vi "Front Panel Tyler.vi"() -> ()   [LabVIEW 2017, in "LD Reading.lvclass"]
uses:
  LD Reading.lvclass
  Reference Channel Intensities.ctl
  Sample Channel Intensities.ctl
  Realtime Output.ctl
  LD Reading.lvclass/LD Reading.ctl
  <vilib>/Analysis/baseanly.llb/Mean (DBL).vi
  <vilib>/Utility/file.llb/Write Delimited Spreadsheet (DBL).vi
  <vilib>/Analysis/NI_AALBase.lvlib
panel:
  out "Data Collection Progress":u8(slide) scale=0.0..100.0
  out "Current Phase":string
  in  "Data graphs":enum32{"Data", "Miscellaneous Data"}(tab)
  out "Diode/PMT":cluster{dbl[], dbl[]}(graph)
  out "RMS Voltage (mV)":cluster{dbl[], dbl[]}(graph)
  out "Photodiode Voltage  (V)":cluster{dbl[], dbl[]}(graph)
  out "PMT Voltage (V)":cluster{dbl[], dbl[]}(graph)
  in  "Data Collection Mode":enum32{"Reference", "Sample"}(radio)
  in  "Selected Sample Channel":enum32{"Channel 1", "Channel 2", "Channel 3"}(radio)
  in  "Selected Reference Channel":enum32{"Channel 1", "Channel 2", "Channel 3"}(radio)
  out "Realtime Output":T1
  out "Sample Data":T2
  out "Reference Data":T3
  in  "Correction Factor":dbl
  out "Finished":bool
  in  "Output Filename (stem)":path
  in  "Stop Data Collection":bool
  in  "Save Data?":bool
  out "Running":bool
  in  "Number of Data Points":dbl
  in  "Data Interval (s)":dbl
  in  "Collect Data":bool
  in  "stop":bool
  # "Data Collection Parameters"
  # "Experiment Control"
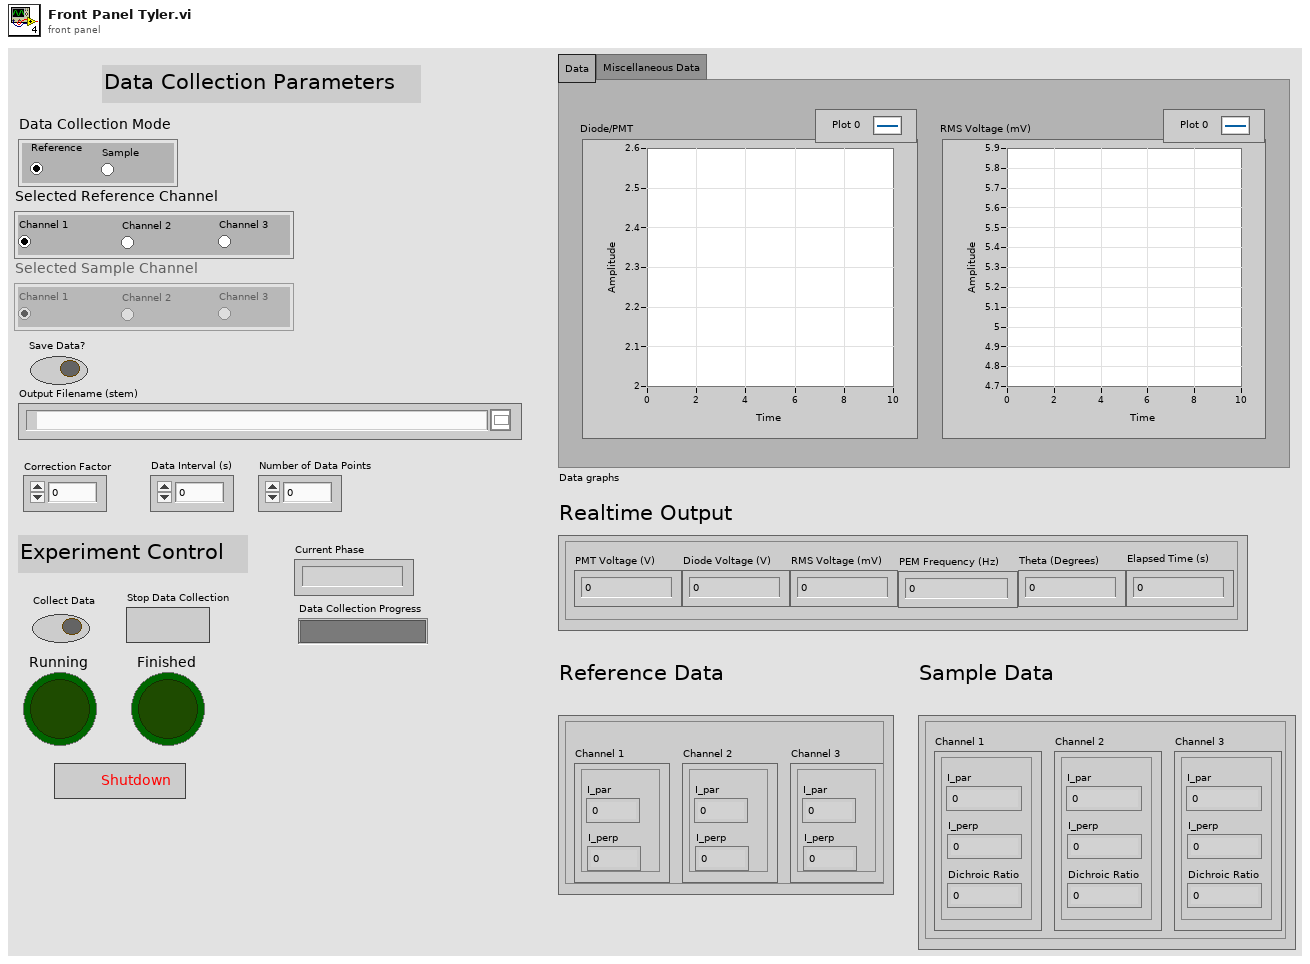
[diagram p1: front panel]
types:
  T1 = typedef "Realtime Output.ctl" = cluster{"Elapsed Time (s)":dbl, "PMT Voltage (V)":dbl, "Diode Voltage (V)":dbl, "RMS Voltage (mV)":dbl, "Theta (Degrees)":dbl, "PEM Frequency (Hz)":dbl}
  T2 = typedef "Sample Channel Intensities.ctl" = cluster{"Channel 1":cluster{"I_par":dbl, "I_perp":dbl, "Dichroic Ratio":dbl}, "Channel 2":cluster{"I_par":dbl, "I_perp":dbl, "Dichroic Ratio":dbl}, "Channel 3":cluster{"I_par":dbl, "I_perp":dbl, "Dichroic Ratio":dbl}}
  T3 = typedef "Reference Channel Intensities.ctl" = cluster{"Channel 1":cluster{"I_par":dbl, "I_perp":dbl}, "Channel 2":cluster{"I_par":dbl, "I_perp":dbl}, "Channel 3":cluster{"I_par":dbl, "I_perp":dbl}}
  T4 = enum8{"Enabled", "Disabled", "Disabled and Grayed Out"}
  T5 = cluster{"I_par":dbl, "I_perp":dbl, "Dichroic Ratio":dbl}
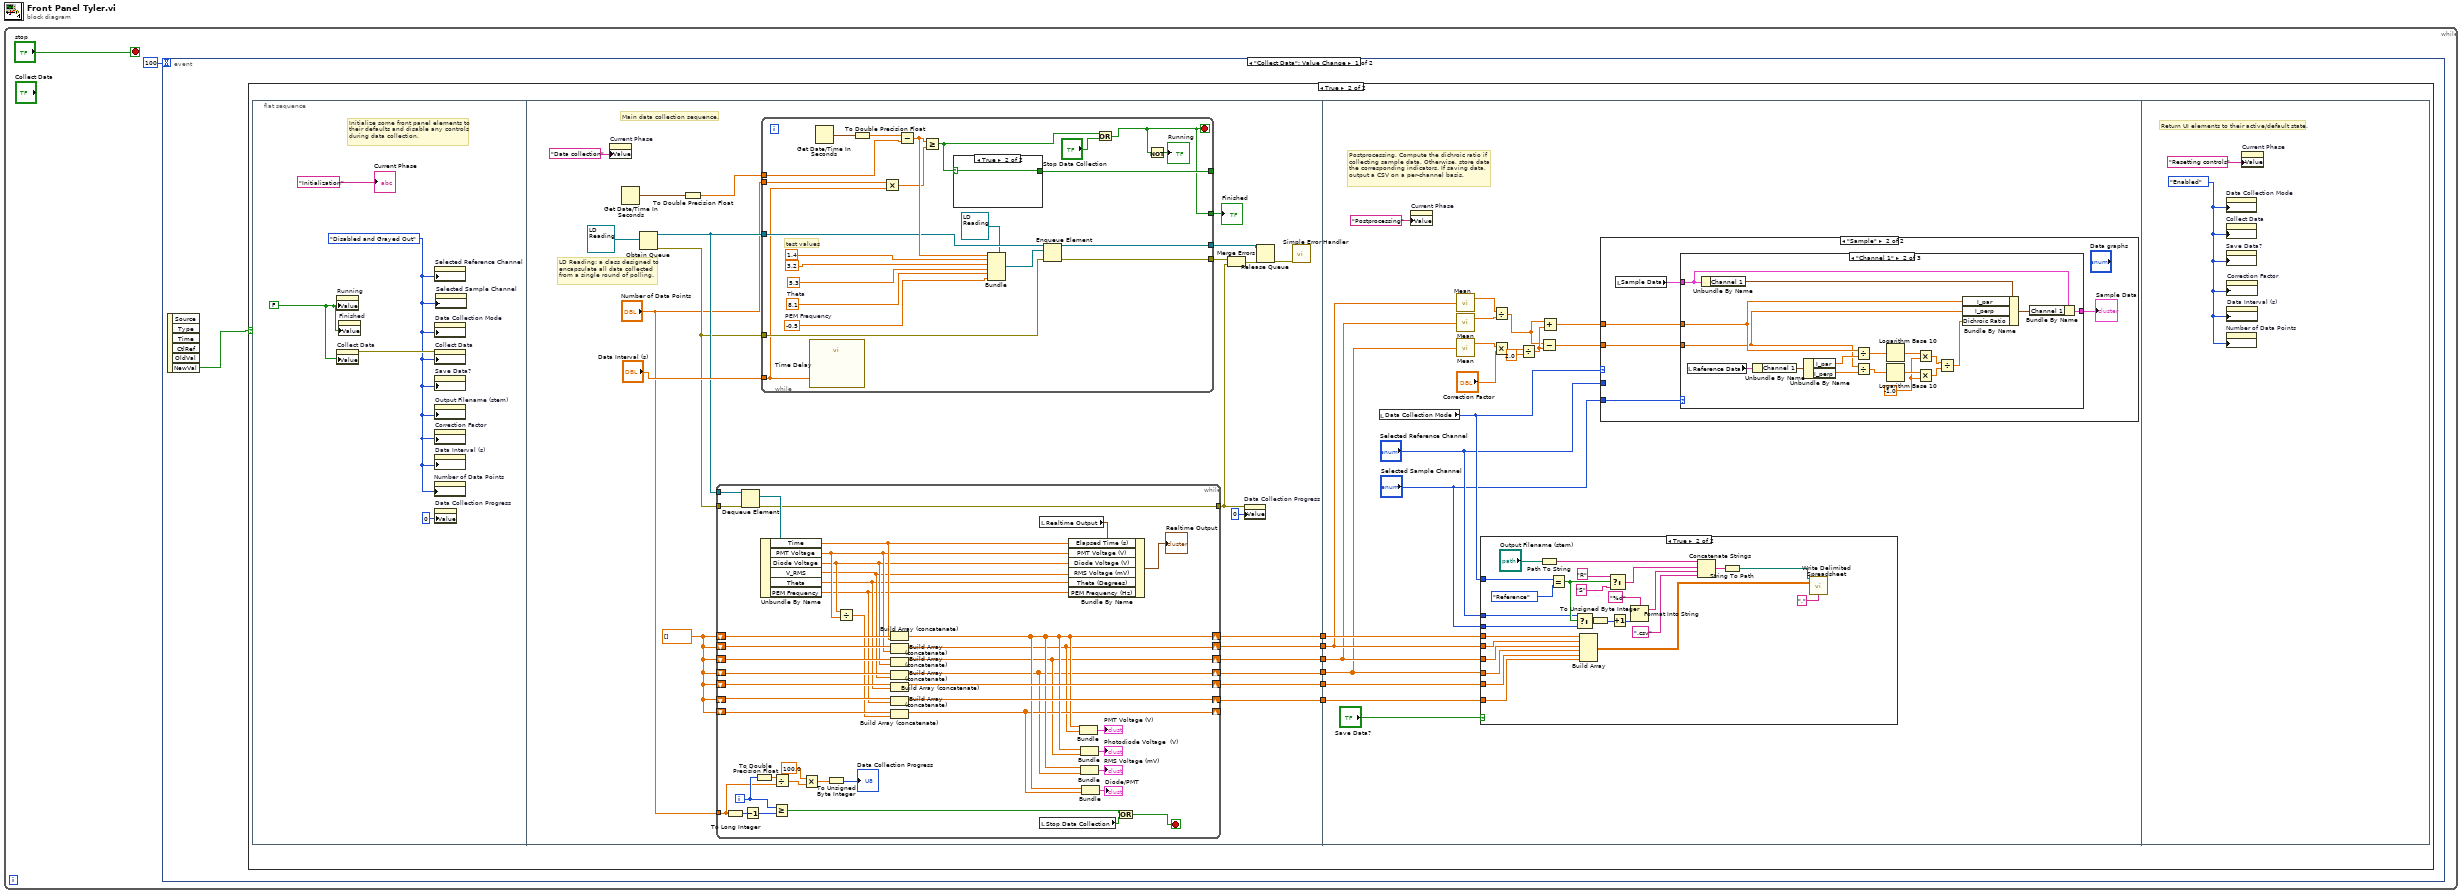
[diagram p0: block diagram]
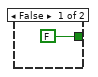
[diagram p3: hidden frame]
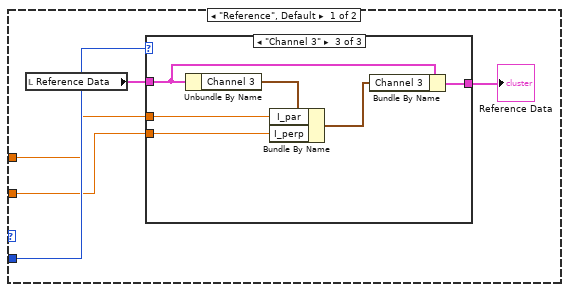
[diagram p5: hidden frame]
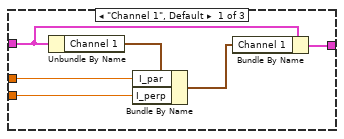
[diagram p6: hidden frame]
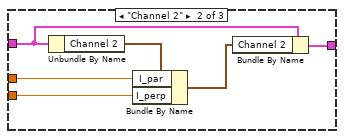
[diagram p7: hidden frame]
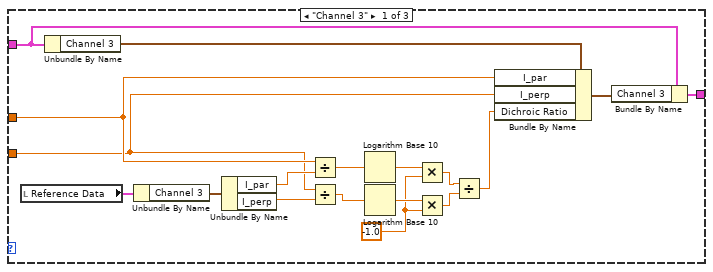
[diagram p8: hidden frame]
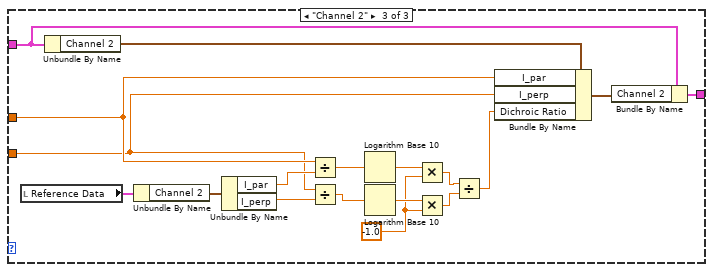
[diagram p9: hidden frame]
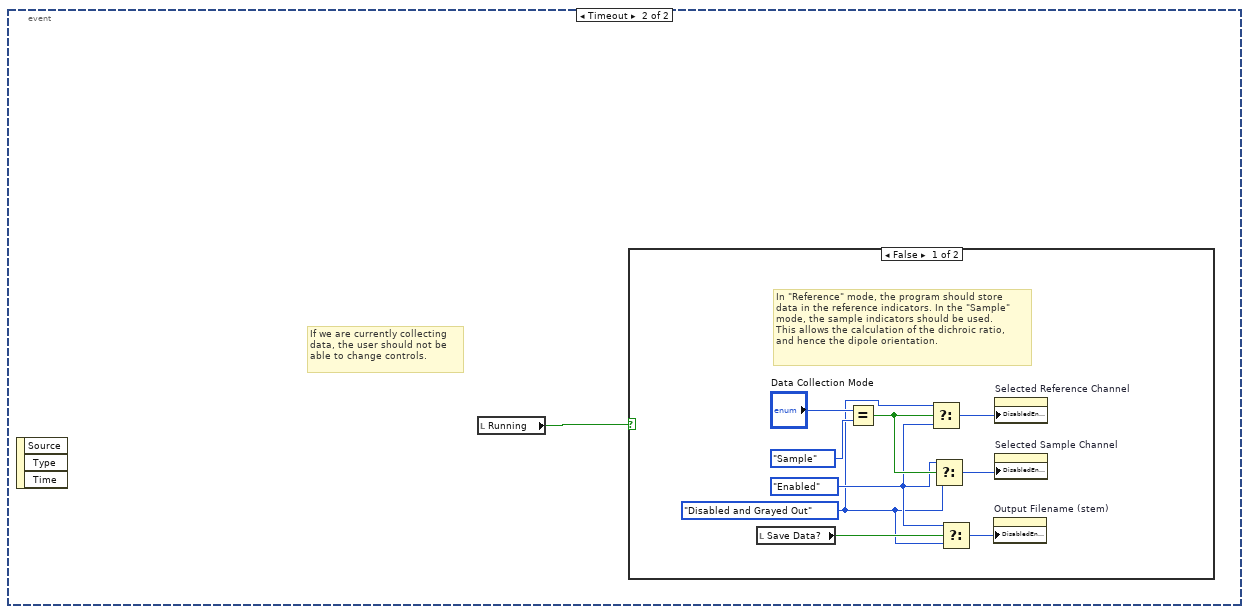
[diagram p10: hidden frame]
diagram:
  n1 = while {
    stop <- "stop" stop-if-true
    n2 = event shown="[0] \"Collect Data\": Value Change" {
      selector: _ -> [_ _]
      dyn-events: _ -> [_ _]
      timeout: 100 -> [_ _]
      event "Collect Data": Value Change {
        n3 = event-data() -> ("NewVal"=w3:bool)  [unwired: 1 in, 5 out]
        n4 = case shown="True" w3 {
          frame False {
          }
          frame True {
            n5 = flat-sequence {
              tunnel: [w23] -> w9
              tunnel: [w22] -> w8
              tunnel: [w21] -> w7
              tunnel: [w24] -> w6
              tunnel: [w20] -> w5
              tunnel: [w19] -> w4
              tunnel: w9 -> [w108]
              tunnel: w8 -> [w107]
              tunnel: w7 -> [w106]
              tunnel: w6 -> [w114]
              tunnel: w5 -> [w110]
              tunnel: w4 -> [w109]
              frame #0 {
                w12 = T4."Disabled and Grayed Out" ("Disabled")
                w14 = FALSE
                # "Initialize some front panel elements to \ntheir defaults and disable any controls \nduring data collection."
                n6 = property on="Running" class="Bool (strict)"("Value"=w14) -> ()  [unwired: 2 in, 2 out]
                n7 = property on="Collect Data" class="Bool (strict)"("Value"=w14) -> (error out=w13:errorcluster)  [unwired: 2 in, 1 out]
                n8 = property on="Finished" class="Bool (strict)"("Value"=w14) -> ()  [unwired: 2 in, 2 out]
                n9 = property on="Number of Data Points" class="DigNum (strict)"("DisabledEnum"=w12) -> ()  [unwired: 2 in, 2 out]
                n10 = property on="Selected Reference Channel" class="RadioBtnsControl (strict)"("DisabledEnum"=w12) -> ()  [unwired: 2 in, 2 out]
                n11 = property on="Data Collection Mode" class="RadioBtnsControl (strict)"("DisabledEnum"=w12) -> ()  [unwired: 2 in, 2 out]
                n12 = property on="Collect Data" class="Bool (strict)"(error in=w13, "DisabledEnum"=w12) -> ()  [unwired: 1 in, 2 out]
                n13 = property on="Save Data?" class="Bool (strict)"("DisabledEnum"=w12) -> ()  [unwired: 2 in, 2 out]
                n14 = property on="Output Filename (stem)" class="Path"("DisabledEnum"=w12) -> ()  [unwired: 2 in, 2 out]
                n15 = property on="Correction Factor" class="DigNum (strict)"("DisabledEnum"=w12) -> ()  [unwired: 2 in, 2 out]
                n16 = property on="Data Interval (s)" class="DigNum (strict)"("DisabledEnum"=w12) -> ()  [unwired: 2 in, 2 out]
                n17 = property on="Data Collection Progress" class="Slide (strict)"("Value"=u8 0 ("Progress")) -> ()  [unwired: 2 in, 2 out]
                n18 = property on="Selected Sample Channel" class="RadioBtnsControl (strict)"("DisabledEnum"=w12) -> ()  [unwired: 2 in, 2 out]
                "Current Phase" <- "Initialization"
              }
              frame #1 {
                w18 = dbl[] []
                # "Main data collection sequence."
                # "LD Reading: a class designed to \nencapsulate all data collected \nfrom a single round of polling."
                n19 = property on="Current Phase" class="Str"("Value"="Data collection") -> ()  [unwired: 2 in, 2 out]
                n20 = Get Date/Time In Seconds() -> (seconds since 1Jan1904=w35:timestamp)
                n21 = Obtain Queue(element data type=refnum<class "LD Reading.lvclass"> refnum ("LD Reading.lvclass")) -> (queue out=w32:refnum<queue>, error out=w30:errorcluster)  [unwired: 4 in, 1 out]
                n22 = To Double Precision Float(number=w35) -> (double precision float=w34:dbl)
                n23 = while {
                  tunnel: w32 -> [w79]
                  shift-right: [w65] -> w24
                  shift-left: w18 -> [w75]
                  shift-right: [w59] -> w23
                  shift-left: w18 -> [w74]
                  shift-right: [w58] -> w22
                  shift-left: w18 -> [w72]
                  shift-right: [w57] -> w21
                  shift-left: w18 -> [w71]
                  shift-right: [w69] -> w20
                  shift-left: w18 -> [w70]
                  shift-right: [w67] -> w19
                  shift-left: w18 -> [w68]
                  shift-right: [w62] -> _
                  shift-left: w18 -> [w64]
                  tunnel: w30 -> [w56]
                  tunnel: [w55] -> w16
                  tunnel: "Number of Data Points" -> [w41]
                  i -> [w42]
                  stop <- w77 stop-if-true
                  n24 = To Long Integer(number=w41) -> (32bit integer=w43:i32)
                  n25 = Dequeue Element(queue=w79, error in (no error)=w56) -> (element=w78:refnum<class "LD Reading.lvclass">, error out=w55:errorcluster)  [unwired: 1 in, 2 out]
                  n26 = Decrement(x=w43) -> (x-1=w54:i32)
                  n27 = To Double Precision Float(number=w42) -> (double precision float=w40:dbl)
                  n28 = Unbundle By Name(w78) -> ("Time"=w51:dbl, "PMT Voltage"=w50:dbl, "Diode Voltage"=w49:dbl, "V_RMS"=w48:dbl, "Theta"=w47:dbl, "PEM Frequency"=w46:dbl)
                  n29 = Greater Or Equal?(x=w42, y=w54) -> (x >= y?=w53:bool)
                  n30 = Divide(x=w40, y=w41) -> (x/y=w44:dbl)
                  n31 = Multiply(x=100.0, y=w44) -> (x*y=w38:dbl)
                  n32 = To Unsigned Byte Integer(number=w38) -> (unsigned 8bit integer=→"Data Collection Progress":u8)
                  n33 = Divide(x=w49, y=w50) -> (x/y=w63:dbl)
                  n34 = Build Array (concatenate)(w75, w51) -> (w65:dbl[])
                  n35 = Build Array (concatenate)(w74, w50) -> (w59:dbl[])
                  n36 = Build Array (concatenate)(w72, w49) -> (w58:dbl[])
                  n37 = Build Array (concatenate)(w71, w48) -> (w57:dbl[])
                  n38 = Build Array (concatenate)(w70, w47) -> (w69:dbl[])
                  n39 = Build Array (concatenate)(w68, w46) -> (w67:dbl[])
                  n40 = Build Array (concatenate)(w64, w63) -> (w62:dbl[])
                  n41 = local read "Realtime Output"() -> (w45:T1)
                  n42 = local read "Stop Data Collection"() -> (w76:bool)
                  n43 = Bundle By Name(cluster=w45, "Elapsed Time (s)"=w51, "PMT Voltage (V)"=w50, "Diode Voltage (V)"=w49, "RMS Voltage (mV)"=w48, "Theta (Degrees)"=w47, "PEM Frequency (Hz)"=w46) -> (→"Realtime Output":T1)
                  n44 = Bundle(w65, w59) -> (→"PMT Voltage (V)":cluster{dbl[], dbl[]})  [unwired: 1 in]
                  n45 = Bundle(w65, w58) -> (→"Photodiode Voltage  (V)":cluster{dbl[], dbl[]})  [unwired: 1 in]
                  n46 = Bundle(w65, w57) -> (→"RMS Voltage (mV)":cluster{dbl[], dbl[]})  [unwired: 1 in]
                  n47 = Bundle(w65, w62) -> (→"Diode/PMT":cluster{dbl[], dbl[]})  [unwired: 1 in]
                  n48 = Or(x=w53, y=w76) -> (x .or. y?=w77:bool)
                }
                n49 = while {
                  tunnel: "Data Interval (s)" -> [w82]
                  tunnel: w34 -> [w83]
                  tunnel: [w99] -> _
                  tunnel: w32 -> [w92]
                  tunnel: [w89] -> w26
                  tunnel: [w86] -> w31
                  tunnel: w30 -> [w85]
                  tunnel: [w84] -> w29
                  tunnel: "Number of Data Points" -> [w81]
                  stop <- w86 stop-if-true
                  w93 = -0.5  # PEM Frequency
                  w94 = 8.1  # Theta
                  # "test values"
                  n50 = call "Time Delay"("Delay Time (s)"=w82) -> ()  [unwired: 10 in, 1 out]
                  n51 = Get Date/Time In Seconds() -> (seconds since 1Jan1904=w102:timestamp)
                  n52 = To Double Precision Float(number=w102) -> (double precision float=w101:dbl)
                  n53 = Multiply(x=w81, y=w82) -> (x*y=w80:dbl)
                  n54 = Subtract(x=w101, y=w83) -> (x-y=w96:dbl)
                  n55 = Greater Or Equal?(x=w96, y=w80) -> (x >= y?=w87:bool)
                  n56 = case shown="True" w87 {
                    selector: w87 -> [_ w104]
                    tunnel: [FALSE w104] -> w99
                    frame False {
                    }
                    frame True {
                    }
                  }
                  n57 = Bundle(cluster=refnum<class "LD Reading.lvclass"> refnum ("LD Reading.lvclass"), w96, 1.4 ("PMT Voltage"), 3.2 ("Diode Voltage"), 5.3 ("V_RMS"), w94, w93) -> (w90:refnum<class "LD Reading.lvclass">)
                  n58 = Enqueue Element(queue=w92, element=w90, error in (no error)=w85) -> (queue out=w89:refnum<queue>, error out=w84:errorcluster)  [unwired: 1 in, 1 out]
                  n59 = Or(x=w87, y="Stop Data Collection") -> (x .or. y?=w86:bool)
                  n60 = Not(x=w86) -> (.not. x?=→"Running":bool)
                }
                "Finished" <- w31
                n61 = Merge Errors(w29, w16) -> (w28:errorcluster)
                n62 = property on="Data Collection Progress" class="Slide (strict)"(error in=w16, "Value"=u8 0 ("Progress")) -> ()  [unwired: 1 in, 2 out]
                n63 = Release Queue(queue=w26, error in (no error)=w28) -> (error out=w27:errorcluster)  [unwired: 1 in, 2 out]
                n64 = call <vilib>:"Simple Error Handler.vi"("error in (no error)"=w27) -> ()  [unwired: 4 in, 5 out]
              }
              frame #2 {
                # "Postprocessing. Compute the dichroic ratio if \ncollecting sample data. Otherwise, store data \nthe corresponding indicators. If saving data, \noutput a CSV on a per-channel basis."
                n65 = local read "Data Collection Mode"() -> (w113:enum32{"Reference", "Sample"})
                n66 = property on="Current Phase" class="Str"("Value"="Postprocessing") -> ()  [unwired: 2 in, 2 out]
                n67 = call-poly <vilib>:"Mean.vi"("X"=w108) -> ("mean"=w118:dbl)  [unwired: 1 out]
                n68 = call-poly <vilib>:"Mean.vi"("X"=w107) -> ("mean"=w117:dbl)  [unwired: 1 out]
                n69 = call-poly <vilib>:"Mean.vi"("X"=w106) -> ("mean"=w124:dbl)  [unwired: 1 out]
                n70 = case shown="True" "Save Data?" {
                  tunnel: w106 -> [_ w133]
                  tunnel: w107 -> [_ w134]
                  tunnel: w108 -> [_ w135]
                  tunnel: w114 -> [_ w136]
                  tunnel: w113 -> [_ w151]
                  tunnel: "Selected Reference Channel" -> [_ w146]
                  tunnel: "Selected Sample Channel" -> [_ w145]
                  tunnel: w110 -> [_ w127]
                  tunnel: w109 -> [_ w126]
                  frame False {
                  }
                  frame True {
                    n71 = Path To String(path="Output Filename (stem)") -> (string=w143:string)
                    n72 = Equal?(x=w151, y=enum32{"Reference", "Sample"}."Reference" ("Data Collection Mode")) -> (x = y?=w147:bool)
                    n73 = Select(t=w146, s=w147, f=w145) -> (s? t:f=w142:enum32{"Channel 1", "Channel 2", "Channel 3"})
                    n74 = Build Array(w136, w135, w134, w133, w127, w126) -> (w132:dbl[][])
                    n75 = To Unsigned Byte Integer(number=w142) -> (unsigned 8bit integer=w130:u8)
                    n76 = Select(t="R", s=w147, f="S") -> (s? t:f=w140:string)
                    n77 = Increment(x=w130) -> (x+1=w129:u8)
                    n78 = Format Into String(format string="%d", w129) -> (resulting string=w139:string)  [unwired: 2 in, 1 out]
                    n79 = Concatenate Strings(w143, w140, w139, ".csv" ("string")) -> (w137:string)
                    n80 = String To Path(string=w137) -> (path=w131:path)
                    n81 = call-poly <vilib>:"Write Delimited Spreadsheet.vi"("file path (dialog if empty)"=w131, "2D data"=w132, "delimiter (\\t)"="," ("delimiter (\\t)")) -> ()  [unwired: 11 in, 2 out]
                  }
                }
                n82 = Divide(x=w118, y=w117) -> (x/y=w116:dbl)
                n83 = Multiply(x=w124, y="Correction Factor") -> (x*y=w123:dbl)
                n84 = Divide(x=w123, y=2.0) -> (x/y=w121:dbl)
                n85 = Subtract(x=w116, y=w121) -> (x-y=w119:dbl)
                n86 = Add(x=w116, y=w121) -> (x+y=w120:dbl)
                n87 = case shown="\"Sample\"" w113 {
                  tunnel: "Selected Reference Channel" -> [w156 _]
                  tunnel: w120 -> [w155 w179]
                  tunnel: w119 -> [w154 w178]
                  tunnel: "Selected Sample Channel" -> [_ w176]
                  frame "Reference", Default {
                    n88 = local read "Reference Data"() -> (w153:T3)
                    n89 = case shown="\"Channel 3\"" w156 {
                      tunnel: w155 -> [w161 w167 w173]
                      tunnel: w154 -> [w160 w166 w172]
                      tunnel: w153 -> [w159 w165 w171]
                      tunnel: [w157 w163 w169] -> w152
                      frame "Channel 1", Default {
                        n90 = Unbundle By Name(w159) -> ("Channel 1"=w162:cluster{"I_par":dbl, "I_perp":dbl})
                        n91 = Bundle By Name(cluster=w162, "I_par"=w161, "I_perp"=w160) -> (w158:cluster{"I_par":dbl, "I_perp":dbl})
                        n92 = Bundle By Name(cluster=w159, "Channel 1"=w158) -> (w157:T3)
                      }
                      frame "Channel 2" {
                        n93 = Unbundle By Name(w165) -> ("Channel 2"=w168:cluster{"I_par":dbl, "I_perp":dbl})
                        n94 = Bundle By Name(cluster=w168, "I_par"=w167, "I_perp"=w166) -> (w164:cluster{"I_par":dbl, "I_perp":dbl})
                        n95 = Bundle By Name(cluster=w165, "Channel 2"=w164) -> (w163:T3)
                      }
                      frame "Channel 3" {
                        n96 = Unbundle By Name(w171) -> ("Channel 3"=w174:cluster{"I_par":dbl, "I_perp":dbl})
                        n97 = Bundle By Name(cluster=w174, "I_par"=w173, "I_perp"=w172) -> (w170:cluster{"I_par":dbl, "I_perp":dbl})
                        n98 = Bundle By Name(cluster=w171, "Channel 3"=w170) -> (w169:T3)
                      }
                    }
                    "Reference Data" <- w152
                  }
                  frame "Sample" {
                    n99 = local read "Sample Data"() -> (w177:T2)
                    n100 = case shown="\"Channel 1\"" w176 {
                      tunnel: w179 -> [w186 w204 w222]
                      tunnel: w178 -> [w185 w203 w221]
                      tunnel: w177 -> [w182 w200 w218]
                      tunnel: [w180 w198 w216] -> w175
                      frame "Channel 3" {
                        w189 = -1.0
                        n101 = local read "Reference Data"() -> (w197:T3)
                        n102 = Unbundle By Name(w182) -> ("Channel 3"=w184:T5)
                        n103 = Unbundle By Name(w197) -> ("Channel 3"=w196:cluster{"I_par":dbl, "I_perp":dbl})
                        n104 = Unbundle By Name(w196) -> ("I_par"=w195:dbl, "I_perp"=w194:dbl)
                        n105 = Divide(x=w186, y=w195) -> (x/y=w192:dbl)
                        n106 = Divide(x=w185, y=w194) -> (x/y=w193:dbl)
                        n107 = Logarithm Base 10(1:w192) -> (0:w190:dbl)
                        n108 = Logarithm Base 10(1:w193) -> (0:w191:dbl)
                        n109 = Multiply(x=w190, y=w189) -> (x*y=w187:dbl)
                        n110 = Multiply(x=w191, y=w189) -> (x*y=w188:dbl)
                        n111 = Divide(x=w187, y=w188) -> (x/y=w183:dbl)
                        n112 = Bundle By Name(cluster=w184, "I_par"=w186, "I_perp"=w185, "Dichroic Ratio"=w183) -> (w181:T5)
                        n113 = Bundle By Name(cluster=w182, "Channel 3"=w181) -> (w180:T2)
                      }
                      frame "Channel 1" {
                        w207 = -1.0
                        n114 = local read "Reference Data"() -> (w215:T3)
                        n115 = Unbundle By Name(w200) -> ("Channel 1"=w202:T5)
                        n116 = Unbundle By Name(w215) -> ("Channel 1"=w214:cluster{"I_par":dbl, "I_perp":dbl})
                        n117 = Unbundle By Name(w214) -> ("I_par"=w213:dbl, "I_perp"=w212:dbl)
                        n118 = Divide(x=w204, y=w213) -> (x/y=w210:dbl)
                        n119 = Divide(x=w203, y=w212) -> (x/y=w211:dbl)
                        n120 = Logarithm Base 10(1:w210) -> (0:w208:dbl)
                        n121 = Logarithm Base 10(1:w211) -> (0:w209:dbl)
                        n122 = Multiply(x=w208, y=w207) -> (x*y=w205:dbl)
                        n123 = Multiply(x=w209, y=w207) -> (x*y=w206:dbl)
                        n124 = Divide(x=w205, y=w206) -> (x/y=w201:dbl)
                        n125 = Bundle By Name(cluster=w202, "I_par"=w204, "I_perp"=w203, "Dichroic Ratio"=w201) -> (w199:T5)
                        n126 = Bundle By Name(cluster=w200, "Channel 1"=w199) -> (w198:T2)
                      }
                      frame "Channel 2" {
                        w225 = -1.0
                        n127 = local read "Reference Data"() -> (w233:T3)
                        n128 = Unbundle By Name(w218) -> ("Channel 2"=w220:T5)
                        n129 = Unbundle By Name(w233) -> ("Channel 2"=w232:cluster{"I_par":dbl, "I_perp":dbl})
                        n130 = Unbundle By Name(w232) -> ("I_par"=w231:dbl, "I_perp"=w230:dbl)
                        n131 = Divide(x=w222, y=w231) -> (x/y=w228:dbl)
                        n132 = Divide(x=w221, y=w230) -> (x/y=w229:dbl)
                        n133 = Logarithm Base 10(1:w228) -> (0:w226:dbl)
                        n134 = Logarithm Base 10(1:w229) -> (0:w227:dbl)
                        n135 = Multiply(x=w226, y=w225) -> (x*y=w223:dbl)
                        n136 = Multiply(x=w227, y=w225) -> (x*y=w224:dbl)
                        n137 = Divide(x=w223, y=w224) -> (x/y=w219:dbl)
                        n138 = Bundle By Name(cluster=w220, "I_par"=w222, "I_perp"=w221, "Dichroic Ratio"=w219) -> (w217:T5)
                        n139 = Bundle By Name(cluster=w218, "Channel 2"=w217) -> (w216:T2)
                      }
                    }
                    "Sample Data" <- w175
                  }
                }
              }
              frame #3 {
                w235 = T4."Enabled" ("Disabled")
                # "Return UI elements to their active/default state."
                n140 = property on="Data Collection Mode" class="RadioBtnsControl (strict)"("DisabledEnum"=w235) -> ()  [unwired: 2 in, 2 out]
                n141 = property on="Collect Data" class="Bool (strict)"("DisabledEnum"=w235) -> ()  [unwired: 2 in, 2 out]
                n142 = property on="Save Data?" class="Bool (strict)"("DisabledEnum"=w235) -> ()  [unwired: 2 in, 2 out]
                n143 = property on="Number of Data Points" class="DigNum (strict)"("DisabledEnum"=w235) -> ()  [unwired: 2 in, 2 out]
                n144 = property on="Correction Factor" class="DigNum (strict)"("DisabledEnum"=w235) -> ()  [unwired: 2 in, 2 out]
                n145 = property on="Data Interval (s)" class="DigNum (strict)"("DisabledEnum"=w235) -> ()  [unwired: 2 in, 2 out]
                n146 = property on="Current Phase" class="Str"("Value"="Resetting controls") -> ()  [unwired: 2 in, 2 out]
              }
            }
          }
        }
      }
      event Timeout {
        # "If we are currently collecting \ndata, the user should not be \nable to change controls."
        n147 = event-data() -> ()  [unwired: 1 in, 3 out]
        n148 = local read "Running"() -> (w236:bool)
        n149 = case shown="False" w236 {
          frame False {
            w237 = T4."Disabled and Grayed Out" ("Disabled")
            w238 = T4."Enabled" ("Disabled")
            # "In \"Reference\" mode, the program should store \ndata in the reference indicators. In the \"Sample\" \nmode, the sample indicators should be used. \nThis allows the calculation of the dichroic ratio, \nand hence the dipole orientation."
            n150 = local read "Save Data?"() -> (w239:bool)
            n151 = Equal?(x="Data Collection Mode", y=enum32{"Reference", "Sample"}."Sample") -> (x = y?=w244:bool)
            n152 = Select(t=w237, s=w244, f=w238) -> (s? t:f=w242:T4)
            n153 = Select(t=w238, s=w244, f=w237) -> (s? t:f=w241:T4)
            n154 = Select(t=w238, s=w239, f=w237) -> (s? t:f=w240:T4)
            n155 = property on="Output Filename (stem)" class="Path"("DisabledEnum"=w240) -> ()  [unwired: 2 in, 2 out]
            n156 = property on="Selected Reference Channel" class="RadioBtnsControl (strict)"("DisabledEnum"=w242) -> ()  [unwired: 2 in, 2 out]
            n157 = property on="Selected Sample Channel" class="RadioBtnsControl (strict)"("DisabledEnum"=w241) -> ()  [unwired: 2 in, 2 out]
          }
          frame True {
          }
        }
      }
    }
  }
